vi "SPCSetParameters_HH.vi"(2 "error in (no error)":errorcluster, 3 "FIFO Settings":T1={"Measurement"={"Binning (ms)"=1.0, "External Trigger Condition"=0, "Stop Condition:"=0, "Stop Count"=0.0, "Buffer Size (Photons)"=1024, "No of Channels"=1, "Ext Latch Delay"=0}, "ADC"={"Binning (HH)"=0, "Dither Range"=0, "Count Increment"=1, "Mode"=0}, "SYNC"={"SYNC ZC Level (mV)"=10.0, "SYNC Freq Divider"=3, "SYNC Holdoff (ps)"=0.0, "SYNC Threshold (mV)"=200.0}, "TAC"={"TAC Range (ns)"=50.0, "TAC Gain"=1, "TAC Offset (%)"=0.0, "TAC Limit Low (%)"=0.0, "TAC Limit High (%)"=100.0}, "Ch 2"={"Ch2 ZC Level (mV)"=10.0, "Ch2 Holdoff (ps)"=0.0, "Ch2 Threshold (mV)"=200.0}, "Ch 3"={"Ch3 ZC Level (mV)"=10.0, "Ch3 Holdoff (ps)"=0.0, "Ch3 Threshold (mV)"=200.0}, "Ch 4"={"Ch4 ZC Level (mV)"=10.0, "Ch4 Holdoff (ps)"=0.0, "Ch4 Threshold (mV)"=200.0}, "Ch1"={"Ch1 ZC Level (mV)"=10.0, "Ch1 Holdoff (ps)"=0.0, "Ch1 Threshold (mV)"=200.0}} {"Ch1"."Ch1 Threshold (mV)" min=0 max=1000 format="%.2f"; "Ch1"."Ch1 Holdoff (ps)" min=-99999 max=99999 format="%.2f"; "Ch1"."Ch1 ZC Level (mV)" min=0 max=40 format="%.2f"; "Ch 4"."Ch4 Threshold (mV)" min=0 max=1000 format="%.2f"; "Ch 4"."Ch4 Holdoff (ps)" min=-99999 max=99999 format="%.2f"; "Ch 4"."Ch4 ZC Level (mV)" min=0 max=40 format="%.2f"; "Ch 3"."Ch3 Threshold (mV)" min=0 max=1000 format="%.2f"; "Ch 3"."Ch3 Holdoff (ps)" min=-99999 max=99999 format="%.2f"; "Ch 3"."Ch3 ZC Level (mV)" min=0 max=40 format="%.2f"; "Ch 2"."Ch2 Threshold (mV)" min=0 max=1000 format="%.2f"; "Ch 2"."Ch2 Holdoff (ps)" min=-99999 max=99999 format="%.2f"; "Ch 2"."Ch2 ZC Level (mV)" min=0 max=40 format="%.2f"; "TAC"."TAC Limit High (%)" min=0 max=100 format="%.2f"; "TAC"."TAC Limit Low (%)" min=0 max=100 format="%.2f"; "TAC"."TAC Offset (%)" min=0 max=100 format="%.2f"; "TAC"."TAC Gain" min=1 max=15 step=1; "TAC"."TAC Range (ns)" min=50 max=2000 format="%.2f"; "SYNC"."SYNC Threshold (mV)" min=0 max=1000 format="%.2f"; "SYNC"."SYNC Holdoff (ps)" min=-99999 max=99999 format="%.2f"; "SYNC"."SYNC Freq Divider" items=["1", "2", "4", "8", "16"]; "SYNC"."SYNC ZC Level (mV)" min=0 max=40 format="%.2f"; "ADC"."Mode" items=["T3"]; "ADC"."Binning (HH)" items=["1", "2", "4", "8", "16", "32", "64", "128", "256", "512", "1024"]; "ADC"."Count Increment" min=1 max=255 step=1; "ADC"."Dither Range" min=0 max=256 step=32; "Measurement"."Ext Latch Delay" min=0 max=255 step=1; "Measurement"."Buffer Size (Photons)" min=512 max=131072 step=512; "Measurement"."Stop Count" format="%.2f"; "Measurement"."Stop Condition:" items=["None", "Photon Count", "Time (s)"]; "Measurement"."External Trigger Condition" max=2 step=1; "Measurement"."No of Channels" max=14; "Measurement"."Binning (ms)" min=1e-07 max=100000 format="%.3f"}) -> (0 "error (out)":errorcluster)   [LabVIEW 2009]
uses:
  FIFOSettings.ctt
panel:
  out "Resolution":dbl
  # "--->"
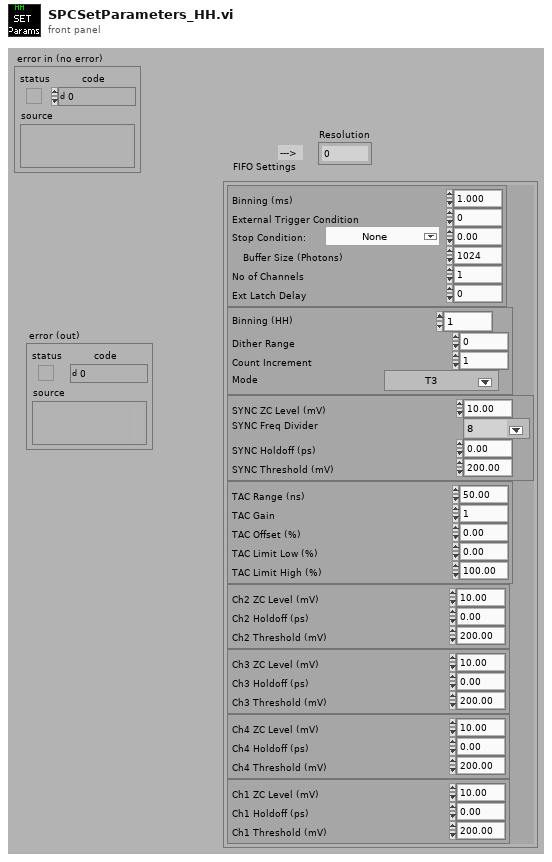
[diagram p1: front panel]
types:
  T1 = typedef "FIFOSettings.ctt" = cluster{"Measurement":cluster{"Binning (ms)":sgl, "External Trigger Condition":u16, "Stop Condition:":u16, "Stop Count":dbl, "Buffer Size (Photons)":u32, "No of Channels":u16, "Ext Latch Delay":i16}, "ADC":cluster{"Binning (HH)":i16, "Dither Range":i16, "Count Increment":i16, "Mode":u16}, "SYNC":cluster{"SYNC ZC Level (mV)":sgl, "SYNC Freq Divider":u16, "SYNC Holdoff (ps)":sgl, "SYNC Threshold (mV)":sgl}, "TAC":cluster{"TAC Range (ns)":sgl, "TAC Gain":i16, "TAC Offset (%)":sgl, "TAC Limit Low (%)":sgl, "TAC Limit High (%)":sgl}, "Ch 2":cluster{"Ch2 ZC Level (mV)":sgl, "Ch2 Holdoff (ps)":sgl, "Ch2 Threshold (mV)":sgl}, "Ch 3":cluster{"Ch3 ZC Level (mV)":sgl, "Ch3 Holdoff (ps)":sgl, "Ch3 Threshold (mV)":sgl}, "Ch 4":cluster{"Ch4 ZC Level (mV)":sgl, "Ch4 Holdoff (ps)":sgl, "Ch4 Threshold (mV)":sgl}, "Ch1":cluster{"Ch1 ZC Level (mV)":sgl, "Ch1 Holdoff (ps)":sgl, "Ch1 Threshold (mV)":sgl}}
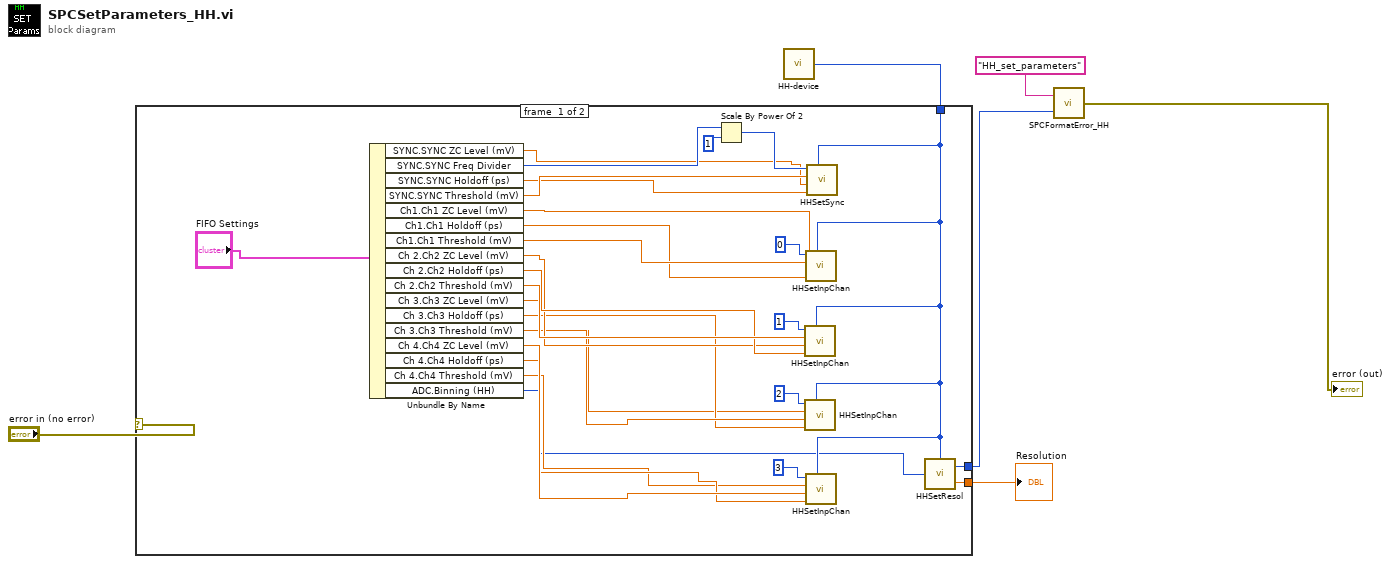
[diagram p0: block diagram]
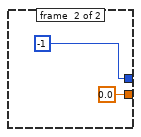
[diagram p2: hidden frame]
diagram:
  n1 = call "HH-device.vi"() -> ("Device (output)"=w5:i32)  [unwired: 2 in]
  n2 = case shown="No Error" "error in (no error)" {
    tunnel: [w27 -1] -> w2
    tunnel: [w26 0.0 ("Resolution")] -> w1
    tunnel: w5 -> [w25 _]
    frame #0 {
      n3 = Unbundle By Name("FIFO Settings") -> ("SYNC.SYNC ZC Level (mV)"=w22:sgl, "SYNC.SYNC Freq Divider"=w24:u16, "SYNC.SYNC Holdoff (ps)"=w21:sgl, "SYNC.SYNC Threshold (mV)"=w23:sgl, "Ch1.Ch1 ZC Level (mV)"=w19:sgl, "Ch1.Ch1 Holdoff (ps)"=w18:sgl, "Ch1.Ch1 Threshold (mV)"=w20:sgl, "Ch 2.Ch2 ZC Level (mV)"=w15:sgl, "Ch 2.Ch2 Holdoff (ps)"=w16:sgl, "Ch 2.Ch2 Threshold (mV)"=w17:sgl, "Ch 3.Ch3 ZC Level (mV)"=w14:sgl, "Ch 3.Ch3 Holdoff (ps)"=w13:sgl, "Ch 3.Ch3 Threshold (mV)"=w12:sgl, "Ch 4.Ch4 ZC Level (mV)"=w11:sgl, "Ch 4.Ch4 Holdoff (ps)"=w10:sgl, "Ch 4.Ch4 Threshold (mV)"=w9:sgl, "ADC.Binning (HH)"=w8:i16)
      n4 = Scale By Power Of 2(n=w24, x=1) -> (x*2^n=w32:i32)
      n5 = call "HHSetInpChan.vi"("Channel"=1, "CFD Level"=w17, "CFD ZeroX"=w15, "Offset"=w16, "DeviceIndex"=w25) -> ()  [unwired: 1 in, 1 out]
      n6 = call "HHSetInpChan.vi"("Channel"=2, "CFD Level"=w12, "CFD ZeroX"=w14, "Offset"=w13, "DeviceIndex"=w25) -> ()  [unwired: 1 in, 1 out]
      n7 = call "HHSetInpChan.vi"("Channel"=0, "CFD Level"=w20, "CFD ZeroX"=w19, "Offset"=w18, "DeviceIndex"=w25) -> ()  [unwired: 1 in, 1 out]
      n8 = call "HHSetInpChan.vi"("Channel"=3, "CFD Level"=w9, "CFD ZeroX"=w11, "Offset"=w10, "DeviceIndex"=w25) -> ()  [unwired: 1 in, 1 out]
      n9 = call "HHSetSync.vi"("SyncDiv"=w32, "CFD Level"=w23, "CFD ZeroX"=w22, "Offset"=w21, "DeviceIndex"=w25) -> ()  [unwired: 1 in, 1 out]
      n10 = call "HHSetResol.vi"("DeviceIndex"=w25, "Binning"=w8) -> ("Resolution"=w26:dbl, "error"=w27:i32)  [unwired: 2 in]
    }
    frame #1 {
    }
  }
  "Resolution" <- w1
  n11 = call "SPCFormatError_HH.vi"("Error Code"=w2, "Source"="HH_set_parameters") -> ("error out"=→"error (out)":errorcluster)
